vi "IDrawable Draw.vi"(7 "Drawing Settings":T1, 8 "error in (no error)":errorcluster, 10 "2D Picture":picture, 11 "Snake in":refnum<class "Snake.lvclass">) -> (0 "error out":errorcluster, 2 "2D Picture out":picture, 3 "Snake out":refnum<class "Snake.lvclass">)   [LabVIEW 2020, in "Snake.lvclass"]
uses:
  Snake.lvclass
  Drawing Settings STYP.ctl
  Snake.lvclass/Snake.ctl
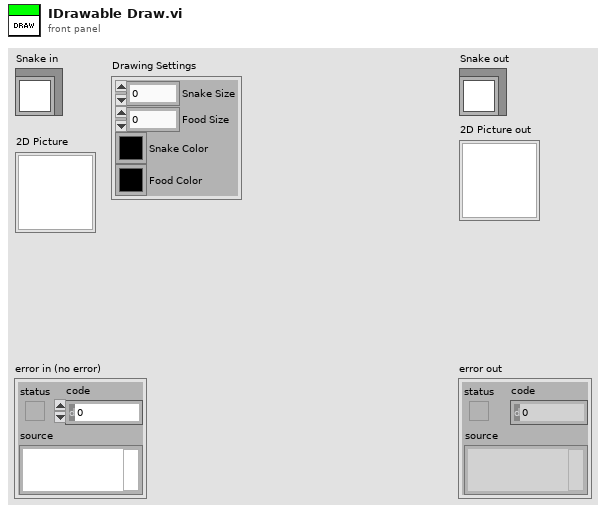
[diagram p1: front panel]
types:
  T1 = typedef "Drawing Settings STYP.ctl" = cluster{"Snake Size":u32, "Food Size":u32, "Snake Color":u32, "Food Color":u32}
  T2 = typedef "Snake.lvclass/Snake Segment STYP.ctl" = cluster{"Location":cluster{"x":u32, "y":u32}, "Direction":T3}
  T3 = typedef "Direction STYP.ctl" = enum16{"Up", "Down", "Left", "Right"}
  T4 = cluster{"left":i16, "top":i16, "right":i16, "bottom":i16}
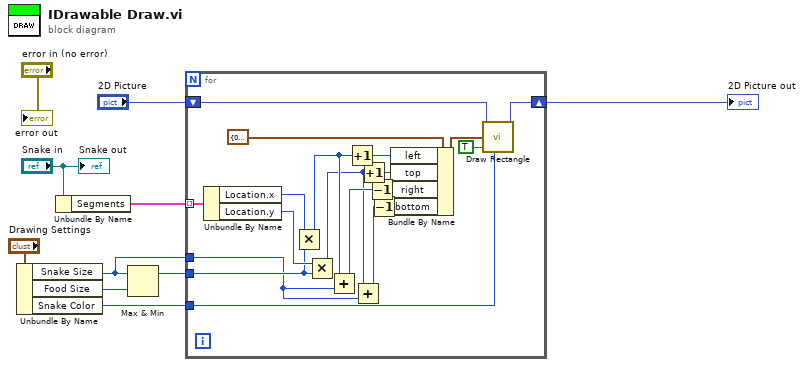
[diagram p0: block diagram]
diagram:
  n1 = Unbundle By Name("Drawing Settings") -> ("Snake Size"=w1:u32, "Food Size"=w4:u32, "Snake Color"=w2:u32)
  n2 = Unbundle By Name("Snake in") -> ("Segments"=w8:T2[])
  n3 = Max & Min(x=w1, y=w4) -> (max(x,y)=w3:u32)  [unwired: 1 out]
  n4 = for {
    tunnel: w8 -> [w23] mode=indexing
    shift-right: [w28] -> w6
    shift-left: "2D Picture" -> [w29]
    tunnel: w3 -> [w20]
    tunnel: w2 -> [w27]
    tunnel: w1 -> [w16]
    n5 = Unbundle By Name(w23) -> ("Location.x"=w22:u32, "Location.y"=w21:u32)
    n6 = Multiply(x=w22, y=w20) -> (x*y=w19:u32)
    n7 = Multiply(x=w21, y=w20) -> (x*y=w17:u32)
    n8 = Add(x=w19, y=w16) -> (x+y=w18:u32)
    n9 = Increment(x=w19) -> (x+1=w14:u32)
    n10 = Add(x=w17, y=w16) -> (x+y=w15:u32)
    n11 = Increment(x=w17) -> (x+1=w13:u32)
    n12 = Decrement(x=w18) -> (x-1=w12:u32)
    n13 = Decrement(x=w15) -> (x-1=w11:u32)
    n14 = Bundle By Name(cluster=T4 {"left"=0, "top"=0, "right"=0, "bottom"=0} ("rect"), "left"=w14, "top"=w13, "right"=w12, "bottom"=w11) -> (w24:T4)
    n15 = call <vilib>:"Draw Rectangle.vi"("picture"=w29, "rect"=w24, "fill?(F)"=TRUE, "color(black)"=w27) -> ("new picture"=w28:picture)  [unwired: 5 in]
  }
  "2D Picture out" <- w6
  "error out" <- "error in (no error)"
  "Snake out" <- "Snake in"
